vi "Windows.DisableAccess.vi"(1 "Enable/Disable":bool) -> ()   [LabVIEW 2019, in "Tools.lvlib"]
uses:
  Tools.lvlib
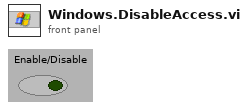
[diagram p1: front panel]
types:
  T1 = enum16{"Show Clock (WIN 9x, NT , 2K, XP )", "Show Taskbar (WIN 9x, NT , 2K, XP )", "Show Start Button (WIN 9x, NT , 2K, XP )", "Show Desktop (WIN 9x, NT , 2K, XP )", "Enable Keys ( Win 9x )", "ALT Tab Enable ( win ? )", "ALT Tab Enable  (WINNT , 2K )", "Enable TaskSwitching  (WINNT , 2K )", "Enable TaskManager (WINNT , 2K )", "Enable CtrlAltDel (WINNT , 2K)"}[]
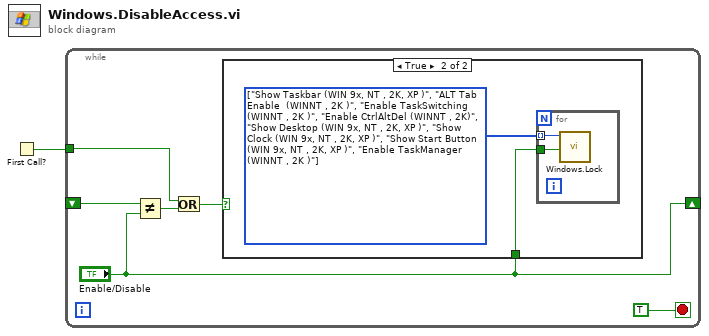
[diagram p0: block diagram]
diagram:
  n1 = First Call?() -> (First Call?: T/F=w1:bool)
  n2 = while {
    shift-right: ["Enable/Disable"] -> _
    shift-left: _ -> [w7]
    tunnel: w1 -> [w5]
    stop <- TRUE stop-if-true
    n3 = Not Equal?(x=w7, y="Enable/Disable") -> (x != y?=w6:bool)
    n4 = Or(x=w5, y=w6) -> (x .or. y?=w4:bool)
    n5 = case shown="True" w4 {
      tunnel: "Enable/Disable" -> [_ w8]
      frame False {
      }
      frame True {
        w9 = T1 [enum."Show Taskbar (WIN 9x, NT , 2K, XP )", enum."ALT Tab Enable  (WINNT , 2K )", enum."Enable TaskSwitching  (WINNT , 2K )", enum."Enable CtrlAltDel (WINNT , 2K)", enum."Show Desktop (WIN 9x, NT , 2K, XP )", enum."Show Clock (WIN 9x, NT , 2K, XP )", enum."Show Start Button (WIN 9x, NT , 2K, XP )", enum."Enable TaskManager (WINNT , 2K )"] items=["Show Clock (WIN 9x, NT , 2K, XP )", "Show Taskbar (WIN 9x, NT , 2K, XP )", "Show Start Button (WIN 9x, NT , 2K, XP )", "Show Desktop (WIN 9x, NT , 2K, XP )", "Enable Keys ( Win 9x )", "ALT Tab Enable ( win ? )", "ALT Tab Enable  (WINNT , 2K )", "Enable TaskSwitching  (WINNT , 2K )", "Enable TaskManager (WINNT , 2K )", "Enable CtrlAltDel (WINNT , 2K)"]
        n6 = for {
          tunnel: w9 -> [w11] mode=indexing
          tunnel: w8 -> [w10]
          n7 = call "Windows.Lock.vi"("Action"=w11, "Show/Enable"=w10) -> ()  [unwired: 18 out]
        }
      }
    }
  }
